vi "LMS_EnableTxWFM.vi"(8 "error in (no error)":errorcluster, 9 "active":i8, 10 "chan":u64, 11 "device_In":i64) -> (0 "error out":errorcluster, 3 "device_Out":i64)   [LabVIEW 2018, in "LMS_LV_Drv.lvlib"]
uses:
  LMS_LV_Drv.lvlib
  C:/Program Files/PothosSDR/bin/LimeSuite.dll
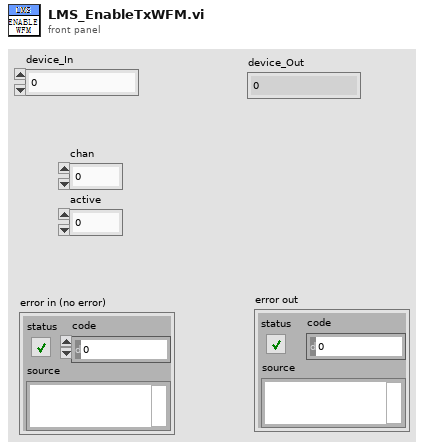
[diagram p1: front panel]
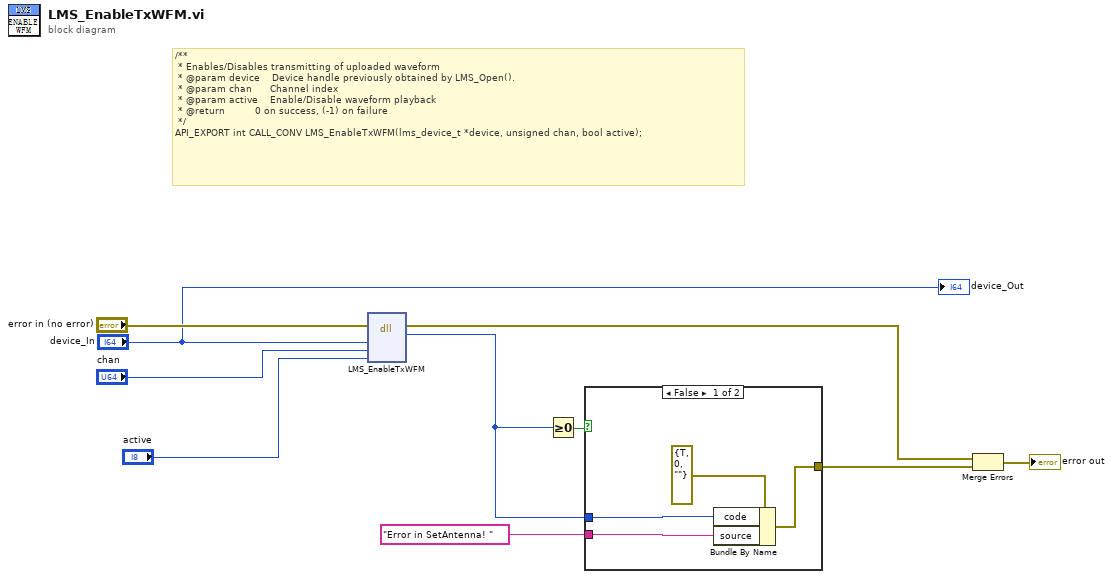
[diagram p0: block diagram]
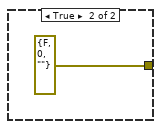
[diagram p2: hidden frame]
diagram:
  # "/**\n * Enables/Disables transmitting of uploaded waveform\n * @param device    Device handle previously obtained by LMS_Open().\n * @param chan      Channel index\n * @param active    Enable/Disable waveform playback\n * @return          0 on success, (-1) on failure\n */\nAPI_EXPORT int CALL_CONV LMS_EnableTxWFM(lms_device_t *device, unsigned chan, bool active);"
  n1 = dll-call lib="C:/Program Files/PothosSDR/bin/LimeSuite.dll" fn="LMS_EnableTxWFM"(error in="error in (no error)", "device"="device_In", "chan"="chan", "active"="active") -> (error out=w4:errorcluster, "return type"=w5:i32)  [unwired: 5 in, 1 out]
  n2 = Greater Or Equal To 0?(x=w5) -> (x >= 0?=w8:bool)
  n3 = case shown="False" w8 {
    tunnel: [w13 errorcluster {"status"=FALSE, "code"=0, "source"=""} ("error in")] -> w6
    tunnel: w5 -> [w12 _]
    tunnel: "Error in SetAntenna! " ("source") -> [w11 _]
    frame False {
      n4 = Bundle By Name(cluster=errorcluster {"status"=TRUE, "code"=0, "source"=""} ("error in"), "code"=w12, "source"=w11) -> (w13:errorcluster)
    }
    frame True {
    }
  }
  n5 = Merge Errors(w4, w6) -> (→"error out":errorcluster)
  "device_Out" <- "device_In"
